vi "LcWebView_Create.vi"(0 "reference in":refnum<class "LcWebView.lvclass">, 1 "Webview container":refnum<k24>(container), 2 "User Data Folder":path, 5 "Error In":errorcluster) -> (12 "BrowserProcessId":u32, 13 "User Data Folder":path, 14 "reference out":refnum<class "LcWebView.lvclass">, 15 "Status":i32(ring)=5 items=["Created", "WaitingForActivation", "WaitingToRun", "Running", "WaitingForChildrenToComplete", "RanToCompletion", "Canceled", "Faulted"], 16 "Status Message":string, 17 "Initialise Loops":i32=1, 18 "Reinstall Runtime":bool, 19 "Error Out":errorcluster)   [LabVIEW 2018, in "LcWebView.lvclass"]
uses:
  LcWebView.lvclass
  ctrls/ErrorCode.ctl
  D:/GitProjects/Public/GitHub/LcWebView/data/Microsoft.Web.WebView2.Core.dll
  data/Microsoft.Web.WebView2.Core.dll
  D:/GitProjects/Public/GitHub/LcWebView/data/Microsoft.Web.WebView2.WinForms.dll
  data/Microsoft.Web.WebView2.WinForms.dll
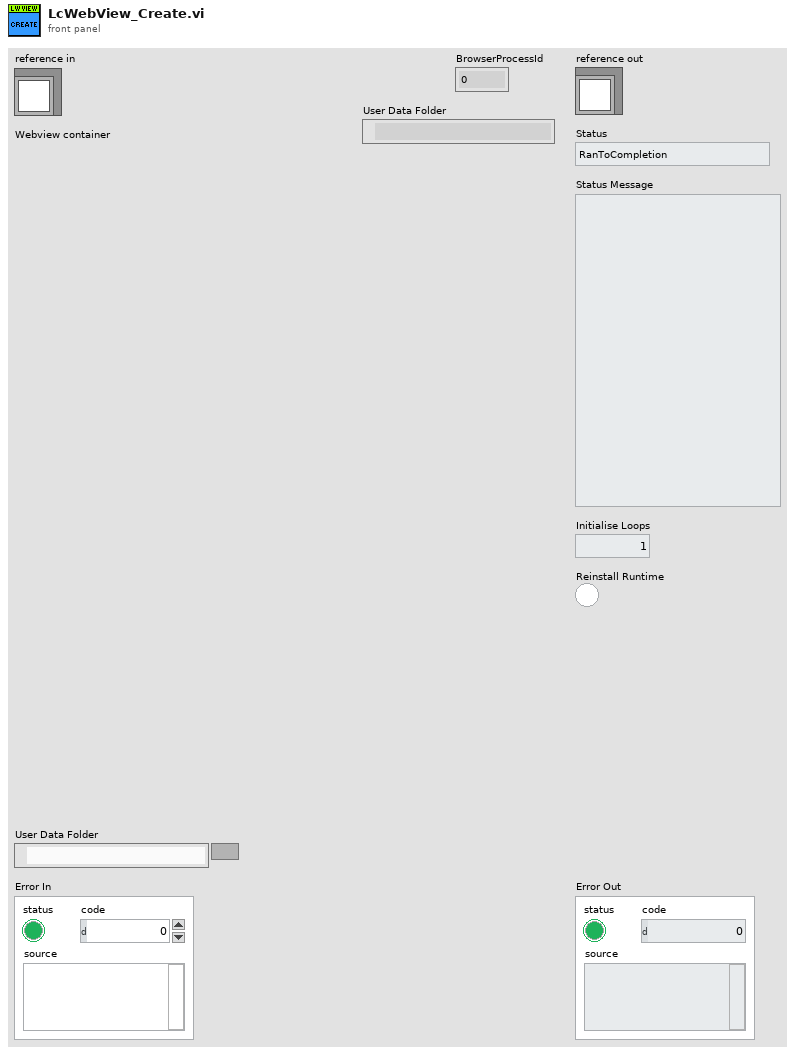
[diagram p1: front panel]
types:
  T1 = typedef "LcWebView.lvclass/ErrorCode.ctl" = enum16{"Runtime engine is not installed or incompatible", "User Data Folder cannot be set", "Others"}
  T2 = typedef "LcWebView.lvclass/ObjectAttributes.ctl" = cluster{"WebView Container":refnum<k24>, "CoreWebViewRef":refnum<k24>, "Status":i32, "Status Message":string, "User Data Folder":path, "BrowserProcessId":u32, "PlotType":T3}
  T3 = typedef "LcWebView.lvclass/PlotType.ctl" = enum16{"bar", "line", "pie", "doughnut", "scatter", "radar", "bubble", "polarArea"}
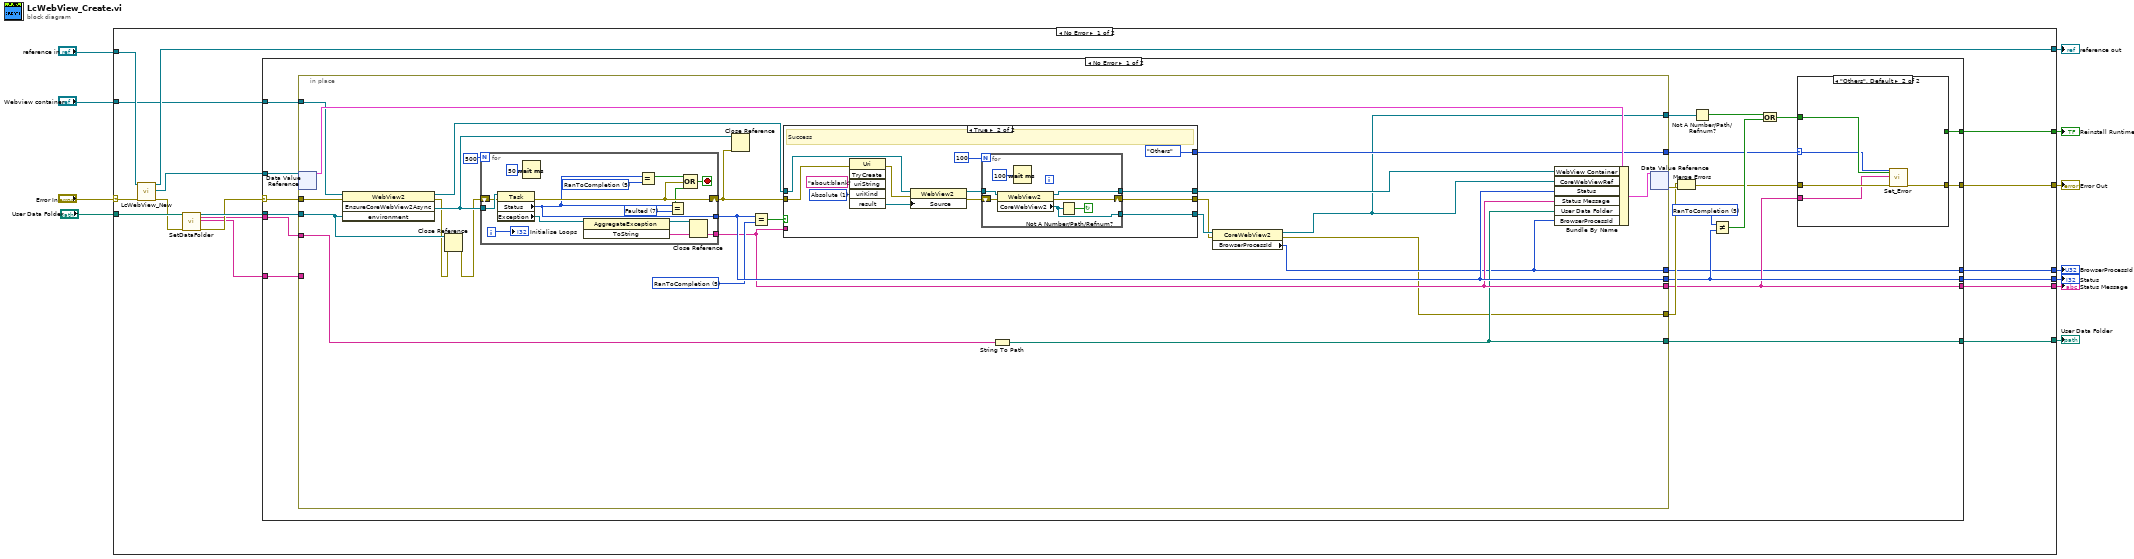
[diagram p0: block diagram]
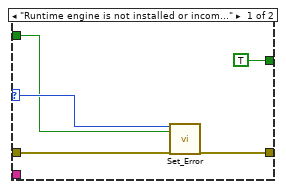
[diagram p2: hidden frame]
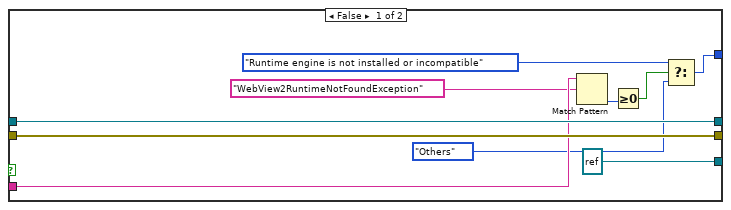
[diagram p3: hidden frame]
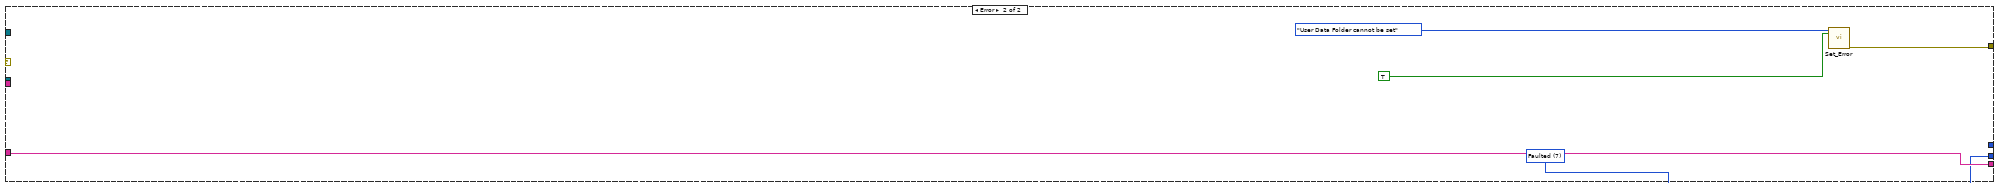
[diagram p4: hidden frame]
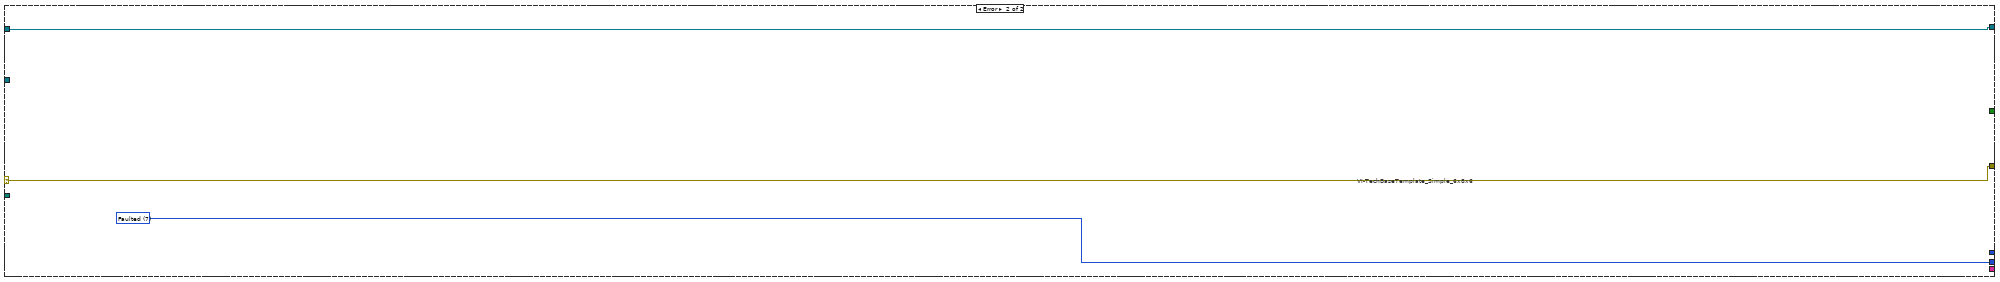
[diagram p5: hidden frame]
diagram:
  n1 = case shown="No Error" "Error In" {
    selector: "Error In" -> [w20 w135]
    tunnel: [w23 w135] -> w10
    tunnel: "reference in" -> [w28 w134]
    tunnel: [w27 w134] -> w8
    tunnel: [w25 w133] -> w7
    tunnel: [w22 _] -> w6
    tunnel: "Webview container" -> [w24 _]
    tunnel: [w21 _] -> w4
    tunnel: "User Data Folder" -> [w19 _]
    tunnel: [w13 _] -> w2
    tunnel: [w12 _] -> w1
    frame No Error {
      n2 = call "LcWebView_New.vi"("reference in"=w28, "error in (no error)"=w20) -> ("reference out"=w27:refnum<class "LcWebView.lvclass">, "DVRRefOut"=w26:refnum<data-value>, "error out"=w16:errorcluster)  [unwired: 14 in, 1 out]
      n3 = call "SetDataFolder.vi"("User Data Folder"=w19, "error in (no error)"=w16) -> ("Environment"=w18:refnum<k24>, "UserDataFolder"=w14:string, "Error Message"=w15:string, "error out"=w17:errorcluster)  [unwired: 14 in]
      n4 = case shown="No Error" w17 {
        selector: w17 -> [w33 _]
        tunnel: w26 -> [w48 _]
        tunnel: [w46 w129] -> w25
        tunnel: w24 -> [w43 _]
        tunnel: [w38 w132] -> w23
        tunnel: [w36 w131] -> w22
        tunnel: [w35 _] -> w21
        tunnel: w18 -> [w34 _]
        tunnel: w15 -> [w32 w131]
        tunnel: w14 -> [w31 _]
        tunnel: [w30 _] -> w13
        tunnel: [w29 _] -> w12
        frame No Error {
          w45 = 5 items=["Created", "WaitingForActivation", "WaitingToRun", "Running", "WaitingForChildrenToComplete", "RanToCompletion", "Canceled", "Faulted"] ("Status")
          n5 = in-place {
            in-place-border: w43 -> [w73]
            in-place-border: [w80] -> w46
            in-place-border: [w75] -> w36
            in-place-border: [w60] -> w47
            in-place-border: [w63] -> w42
            in-place-border: [w74] -> w37
            in-place-border: w34 -> [w67]
            in-place-border: w33 -> [w70]
            in-place-border: w32 -> [_]
            in-place-border: w31 -> [w69]
            in-place-border: [w68] -> w30
            in-place-border: [w61] -> w29
            w79 = 5 items=["Created", "WaitingForActivation", "WaitingToRun", "Running", "WaitingForChildrenToComplete", "RanToCompletion", "Canceled", "Faulted"] ("Status")
            n6 = in-place-dvr #1(w48) -> (w82:T2)  [unwired: 1 out]
            n7 = invoke class="WebView2" method="EnsureCoreWebView2Async"(reference=w73, error in=w70, "environment"=w67) -> (reference out=w71:refnum<k24>, error out=w66:errorcluster, "EnsureCoreWebView2Async"=w77:refnum<k24>)  [unwired: 1 in, 1 out]
            n8 = Close Reference(reference=w67, error in (no error)=w66) -> (error out=w65:errorcluster)
            n9 = for {
              N: 500 -> [_]
              tunnel: w77 -> [w127]
              shift-right: [w120] -> w76
              shift-left: w65 -> [w126]
              tunnel: [w117] -> w80
              tunnel: [w123] -> w75
              i -> [w115]
              stop <- w118 stop-if-true
              w122 = 5 items=["Created", "WaitingForActivation", "WaitingToRun", "Running", "WaitingForChildrenToComplete", "RanToCompletion", "Canceled", "Faulted"] ("Status")
              w124 = 7 items=["Created", "WaitingForActivation", "WaitingToRun", "Running", "WaitingForChildrenToComplete", "RanToCompletion", "Canceled", "Faulted"] ("Status")
              n10 = property class="Task"(reference=w127, error in=w126) -> (error out=w120:errorcluster, "Status"=w117:i32, "Exception"=w125:refnum<k24>)  [unwired: 1 out]
              n11 = Wait (ms)(milliseconds to wait=u32 50) -> ()  [unwired: 1 out]
              n12 = invoke class="AggregateException" method="ToString"(reference=w125) -> (reference out=w116:refnum<k24>, "ToString"=w123:string)  [unwired: 2 in, 1 out]
              n13 = Equal?(x=w117, y=w122) -> (x = y?=w121:bool)
              n14 = Equal?(x=w117, y=w124) -> (x = y?=w119:bool)
              n15 = Compound Arithmetic op=OR(w121, w120, w119) -> (w118:bool)
              n16 = Close Reference(reference=w116) -> ()  [unwired: 1 in, 1 out]
              "Initialise Loops" <- w115
            }
            n17 = Close Reference(reference=w77, error in (no error)=w76) -> ()  [unwired: 1 out]
            n18 = Equal?(x=w80, y=w79) -> (x = y?=w78:bool)
            n19 = case shown="True" w78 {
              tunnel: w76 -> [w91 w98]
              tunnel: [w93 w106] -> w72
              tunnel: [refnum<k24> refnum ("CoreWebView2") w105] -> w64
              tunnel: [w91 w104] -> w62
              tunnel: w71 -> [w93 w97]
              tunnel: w75 -> [w90 _]
              tunnel: [w84 ErrorCode."Others" ("f")] -> w74
              frame False {
                n20 = Match Pattern(string=w90, regular expression="WebView2RuntimeNotFoundException") -> (offset past match=w88:i32)  [unwired: 1 in, 3 out]
                n21 = Greater Or Equal To 0?(x=w88) -> (x >= 0?=w87:bool)
                n22 = Select(t=ErrorCode."Runtime engine is not installed or incompatible" ("CustomErrors"), s=w87, f=ErrorCode."Others") -> (s? t:f=w84:T1)
              }
              frame True {
                w100 = 1 items=["RelativeOrAbsolute", "Absolute", "Relative"] ("uriKind")
                # "Success"
                n23 = invoke class="Uri" method="TryCreate"(error in=w98, "uriString"="about:blank", "uriKind"=w100) -> (error out=w95:errorcluster, "result"=w99:refnum<k24>)  [unwired: 3 in, 4 out]
                n24 = property class="WebView2"(reference=w97, error in=w95, "Source"=w99) -> (reference out=w96:refnum<k24>, error out=w94:errorcluster)
                n25 = for {
                  N: 100 -> [_]
                  tunnel: w96 -> [w113]
                  shift-right: [w110] -> w104
                  shift-left: w94 -> [w111]
                  tunnel: [w108] -> w105
                  tunnel: [w107] -> w106
                  stop <- w109 continue-if-true
                  n26 = property class="WebView2"(reference=w113, error in=w111) -> (reference out=w107:refnum<k24>, error out=w110:errorcluster, "CoreWebView2"=w108:refnum<k24>)
                  n27 = Wait (ms)(milliseconds to wait=u32 100) -> ()  [unwired: 1 out]
                  n28 = Not A Number/Path/Refnum?(number/path/refnum=w108) -> (NaN/Path/Refnum?=w109:bool)
                }
              }
            }
            n29 = String To Path(string=w69) -> (path=w68:path)
            n30 = property class="CoreWebView2"(reference=w64, error in=w62) -> (reference out=w63:refnum<k24>, error out=w60:errorcluster, "BrowserProcessId"=w61:u32)
            n31 = Bundle By Name(cluster=w82, "WebView Container"=w72, "CoreWebViewRef"=w63, "Status"=w80, "Status Message"=w75, "User Data Folder"=w68, "BrowserProcessId"=w61) -> (w83:T2)
            n32 = in-place-dvr #1(w83) -> (w49:errorcluster)  [unwired: 1 out]
          }
          n33 = Merge Errors(w47, w49) -> (w40:errorcluster)
          n34 = Not A Number/Path/Refnum?(number/path/refnum=w42) -> (NaN/Path/Refnum?=w41:bool)
          n35 = Not Equal?(x=w45, y=w46) -> (x != y?=w44:bool)
          n36 = Compound Arithmetic op=OR(w41, w44) -> (w39:bool)
          n37 = case shown="\"Others\", Default" w37 {
            selector: w37 -> [w52 w56]
            tunnel: w40 -> [w54 w59]
            tunnel: w39 -> [w51 w58]
            tunnel: [w53 w57] -> w38
            tunnel: w36 -> [_ w55]
            tunnel: [TRUE _] -> w35
            frame "Runtime engine is not installed or incompatible" {
              n38 = call "Set_Error.vi"("CustomErrors"=w52, "SetError(True)"=w51, "error in (no error)"=w54) -> ("error out"=w53:errorcluster)  [unwired: 16 in]
            }
            frame "Others", Default {
              n39 = call "Set_Error.vi"("CustomErrors"=w56, "SetError(True)"=w58, "Description"=w55, "error in (no error)"=w59) -> ("error out"=w57:errorcluster)  [unwired: 15 in]
            }
          }
        }
        frame Error {
          w129 = 7 items=["Created", "WaitingForActivation", "WaitingToRun", "Running", "WaitingForChildrenToComplete", "RanToCompletion", "Canceled", "Faulted"] ("Status")
          n40 = call "Set_Error.vi"("CustomErrors"=ErrorCode."User Data Folder cannot be set", "SetError(True)"=TRUE) -> ("error out"=w132:errorcluster)  [unwired: 17 in]
        }
      }
    }
    frame Error {
      w133 = 7 items=["Created", "WaitingForActivation", "WaitingToRun", "Running", "WaitingForChildrenToComplete", "RanToCompletion", "Canceled", "Faulted"] ("Status")
      # "VI-TechBaseTemplate_Simple_6x8x6"
    }
  }
  "Error Out" <- w10
  "reference out" <- w8
  "Status" <- w7
  "Status Message" <- w6
  "Reinstall Runtime" <- w4
  "User Data Folder" <- w2
  "BrowserProcessId" <- w1
